vi "Test Internal Oscillator.vi"(8 "error in (no error)":errorcluster, 11 "VISA resource name":refnum<visa-resource-name>) -> (0 "error out":errorcluster, 3 "VISA resource name":refnum<visa-resource-name>)   [LabVIEW 2019, in "SR7270 Drivers.lvlib"]
uses:
  SR7270 Drivers.lvlib
  <vilib>/addons/_JKI Toolkits/Caraya/classes/Test/Test.lvclass
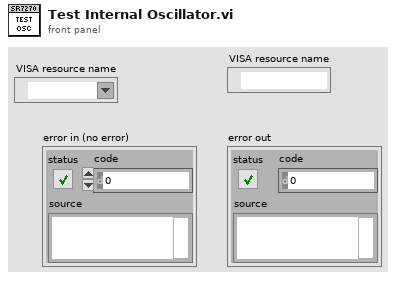
[diagram p1: front panel]
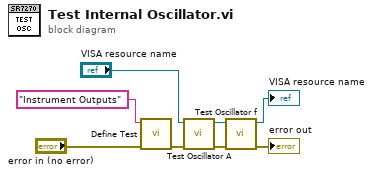
[diagram p0: block diagram]
diagram:
  n1 = call <vilib>:"Define Test.vi"("error in (no error)"="error in (no error)", "Label (VI Title)"="Instrument Outputs") -> ("error out"=w6:errorcluster)  [unwired: 9 in]
  n2 = call "Test Oscillator A.vi"("error in (no error)"=w6, "VISA resource name"="VISA resource name") -> ("error out"=w4:errorcluster, "VISA resource name"=w5:refnum<visa-resource-name>)  [unwired: 8 in]
  n3 = call "Test Oscillator f.vi"("error in (no error)"=w4, "VISA resource name"=w5) -> ("error out"=→"error out":errorcluster, "VISA resource name"=→"VISA resource name":refnum<visa-resource-name>)  [unwired: 8 in]
